vi "testItemLastElement.vi"(8 "error in (no error)":errorcluster, 11 "TestCase in":refnum<class "ListImp_Populated.lvclass">) -> (0 "error out":errorcluster, 3 "TestCase out":refnum<class "ListImp_Populated.lvclass">)   [LabVIEW 2013, in "ListImp_Populated.lvclass"]
uses:
  ListImp_Populated.lvclass
  ListImp_Populated.lvclass/ListImp_Populated.ctl
  source/LapDog.Collections.Lists/ListImp/ListImp.lvclass
  <vilib>/addons/_JKI Toolkits/VI Tester/TestCase.llb/TestCase.lvclass
  UnitTestComparisons/UnitTestComparisons.lvlib
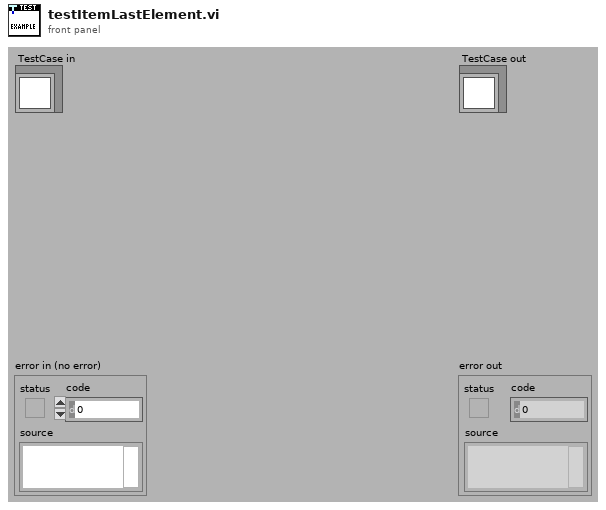
[diagram p1: front panel]
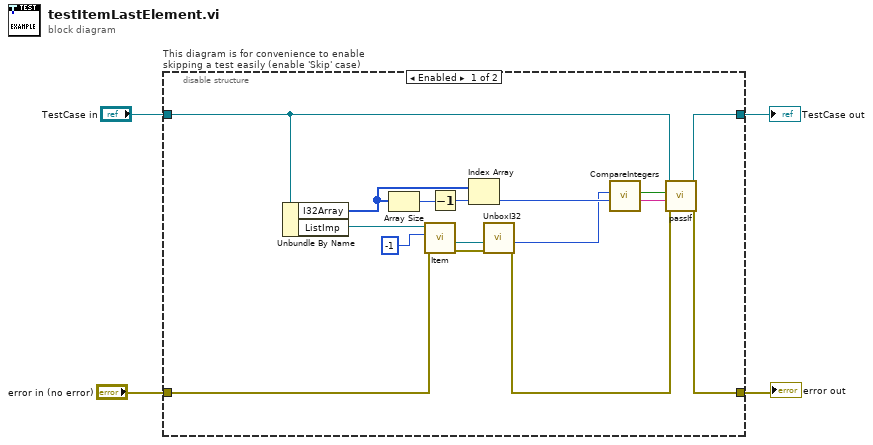
[diagram p0: block diagram]
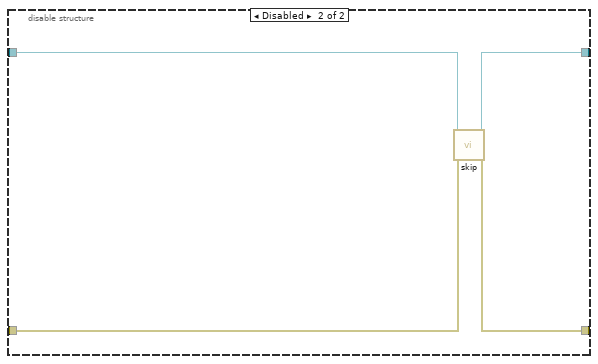
[diagram p2: hidden frame]
diagram:
  n1 = disable-structure "This diagram is for convenience to enable skipping a test easily (enable 'Skip' case)" shown="Enabled" {
    disable-tunnel: "TestCase in" -> [w18 w24]
    disable-tunnel: [w20 w22] -> w1
    disable-tunnel: [w19 w23] -> w3
    disable-tunnel: "error in (no error)" -> [w13 w21]
    frame Enabled {
      n2 = Unbundle By Name(w18) -> ("I32Array"=w12:i32[], "ListImp"=w15:refnum<class "ListImp.lvclass">)
      n3 = Array Size(array=w12) -> (size(s)=w11:i32)
      n4 = call-dynamic "Item.vi"("error in (no error)"=w13, "Index"=-1, "ListImp in"=w15) -> ("error out"=w7:errorcluster, "Item"=w8:refnum<class>)  [unwired: 6 in, 1 out]
      n5 = Decrement(x=w11) -> (x-1=w10:i32)
      n6 = Index Array(array=w12, index=w10) -> (element=w9:i32)
      n7 = call "UnboxI32.vi"("error in (no error)"=w7, "Item"=w8) -> ("error out"=w6:errorcluster, "Value"=w5:i32)  [unwired: 8 in]
      n8 = call "CompareIntegers.vi"("Expected Value"=w9, "Actual Value"=w5) -> ("Message"=w16:string, "Equal?"=w17:bool)  [unwired: 8 in]
      n9 = call-dynamic "passIf.vi"("error in (no error)"=w6, "message (\"\")"=w16, "pass"=w17, "TestCase in"=w18) -> ("error out"=w19:errorcluster, "TestCase out"=w20:refnum<class "ListImp_Populated.lvclass">)  [unwired: 6 in]
    }
    frame Disabled {
      # "skip test result while test is under development"
      n10 = call <vilib>:"skip.vi"("error in (no error)"=w21, "TestCase in"=w24) -> ("error out"=w23:errorcluster, "TestCase out"=w22:refnum<class "ListImp_Populated.lvclass">)  [unwired: 8 in]
    }
  }
  "error out" <- w3
  "TestCase out" <- w1
